vi "ILABs_CreateFromTemplate2.vi"(3 "templatePath":string, 4 "appRef":refnum<vi>) -> ()   [LabVIEW 2009]
panel:
  out "viName":string
  out "viReference":refnum<vi>
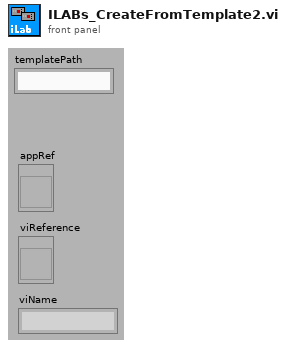
[diagram p1: front panel]
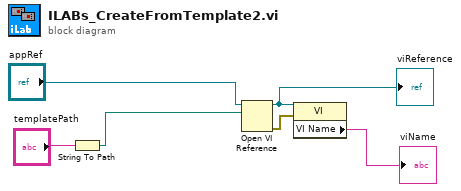
[diagram p0: block diagram]
diagram:
  n1 = String To Path(string="templatePath") -> (path=w3:path)
  n2 = Open VI Reference(application reference (local)="appRef", vi path=w3) -> (vi reference=w6:refnum<vi>, error out=w5:errorcluster)  [unwired: 1 in, 3 out]
  "viReference" <- w6
  n3 = property class="VI"(reference=w6, error in=w5) -> ("VI Name"=→"viName":string)  [unwired: 2 out]
